vi "Check_Conn-s_bet-n_Displ_in_Track_Group-2.vi"(4 "error IN":errorcluster, 5 "[IN] # of Unconne\ncted Problem points":i32, 6 "[IN] #of Frames":i32, 7 "[IN] Clusters for Re\nconstructed Tracks":T1) -> (0 "error OUT":errorcluster, 1 "[OUT] # of Unconne\ncted Problem points":i32, 3 "[OUT] Clusters for Re\nconstructed Tracks":T1)   [LabVIEW 2017]
doc: "This subVI corrects sometimes appearing inaccuracy: appearing of points signed as problem ones but haven't any other connected points with they. The subVI just decrease of statuses of such points"
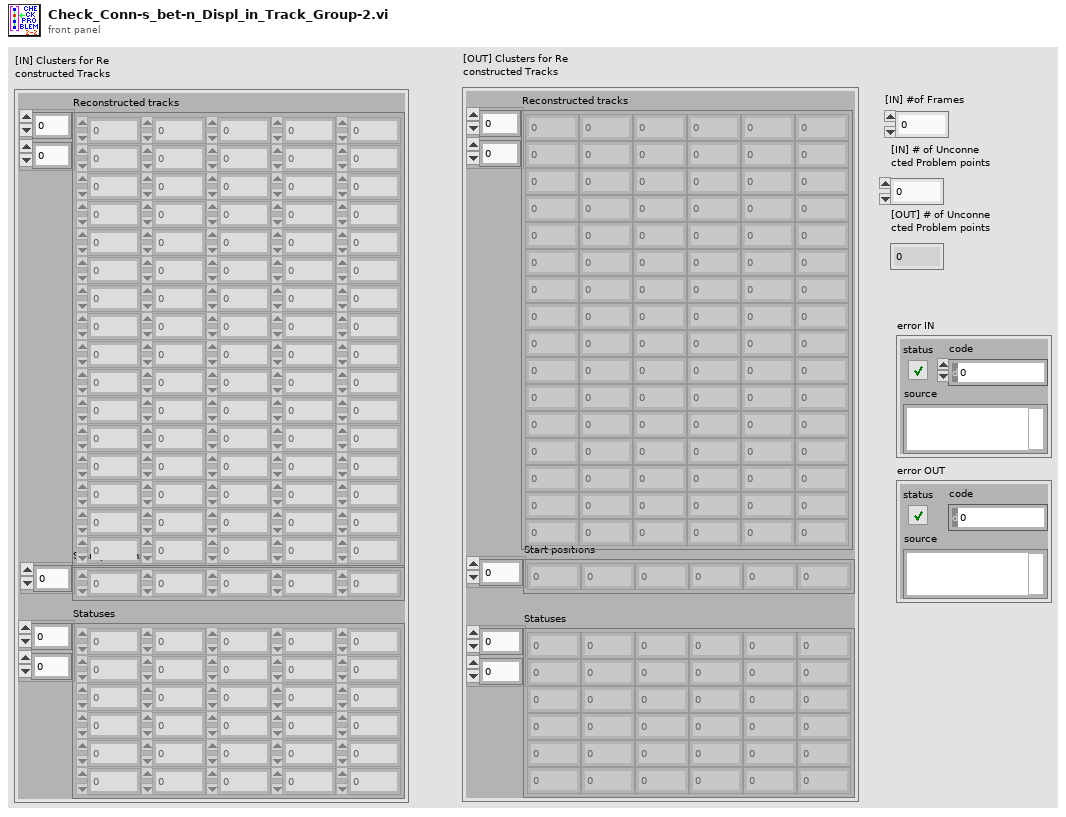
[diagram p1: front panel]
types:
  T1 = cluster{"Reconstructed tracks":dbl[][], "Start positions":i32[], "Statuses":i16[][]}
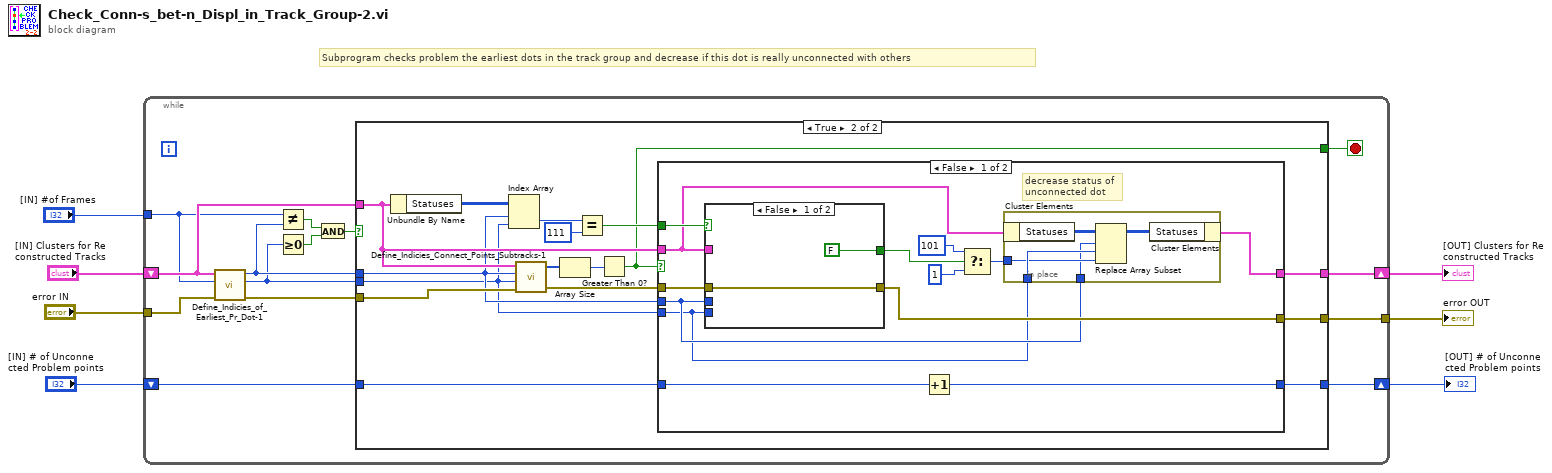
[diagram p0: block diagram]
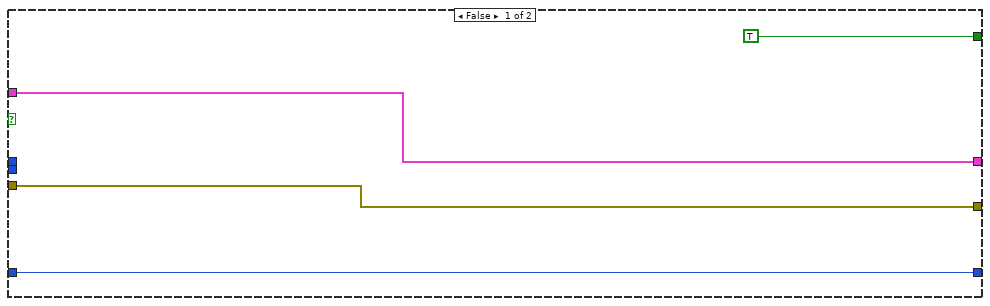
[diagram p2: hidden frame]
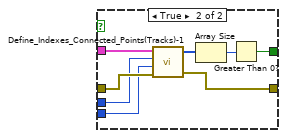
[diagram p3: hidden frame]
diagram:
  # "Subprogram checks problem the earliest dots in the track group and decrease if this dot is really unconnected with others"
  n1 = while {
    shift-right: [w17] -> w3
    shift-left: "[IN] Clusters for Re\nconstructed Tracks" -> [w18]
    tunnel: "error IN" -> [w21]
    shift-right: [w16] -> w5
    shift-left: "[IN] # of Unconne\ncted Problem points" -> [w19]
    tunnel: "[IN] #of Frames" -> [w14]
    tunnel: [w15] -> w1
    stop <- w8 stop-if-true
    n2 = call "Define_Indicies_of_Earliest_Pr_Dot-1.vi"("error IN"=w21, "[IN] #of Frames"=w14, "[IN] Still connected\ntracks in group"=w18) -> ("error OUT"=w20:errorcluster, "[OUT] Index of Subtrack"=w12:i32, "[OUT] Index of Ear\nliest Problem Point"=w13:i32)  [unwired: 2 in]
    n3 = Not Equal?(x=w14, y=w13) -> (x != y?=w10:bool)
    n4 = Greater Or Equal To 0?(x=w12) -> (x >= 0?=w9:bool)
    n5 = And(x=w10, y=w9) -> (x .and. y?=w11:bool)
    n6 = case shown="True" w11 {
      tunnel: w20 -> [w25 w41]
      tunnel: w19 -> [w24 w40]
      tunnel: w18 -> [w23 w39]
      tunnel: w13 -> [_ w37]
      tunnel: w12 -> [_ w36]
      tunnel: [w23 w29] -> w17
      tunnel: [w24 w28] -> w16
      tunnel: [w25 w27] -> w15
      tunnel: [TRUE w26] -> w8
      frame False {
      }
      frame True {
        n7 = Unbundle By Name(w39) -> ("Statuses"=w38:i16[][])
        n8 = Index Array(array=w38, index (row)=w37, index (col)=w36) -> (element=w35:i16)
        n9 = call "Define_Indicies_Connect_Points_Subtracks-1.vi"("error IN"=w41, "[IN] Index of track with\n(problem displacement)"=w36, "[IN] Index of problem\ndisplacement inside track"=w37, "[IN] Track group"=w39) -> ("error OUT"=w32:errorcluster, "[OUT] Index of connected\ntracks with problem dot"=w33:i32[])  [unwired: 1 out]
        n10 = Array Size(array=w33) -> (size(s)=w34:i32)
        n11 = Equal?(x=w35, y=i16 111) -> (x = y?=w30:bool)
        n12 = Greater Than 0?(x=w34) -> (x > 0?=w26:bool)
        n13 = case shown="False" w26 {
          tunnel: w39 -> [w46 w72]
          tunnel: [w45 w72] -> w29
          tunnel: w40 -> [w48 w70]
          tunnel: [w47 w70] -> w28
          tunnel: w37 -> [w43 _]
          tunnel: w36 -> [w42 _]
          tunnel: w32 -> [w53 w71]
          tunnel: [w52 w71] -> w27
          tunnel: w30 -> [w54 _]
          frame False {
            # "decrease status of \nunconnected dot"
            n14 = case shown="False" w54 {
              tunnel: w46 -> [_ w69]
              tunnel: w53 -> [w60 w68]
              tunnel: w43 -> [_ w67]
              tunnel: w42 -> [_ w66]
              tunnel: [FALSE w63] -> w51
              tunnel: [w60 w62] -> w52
              frame False {
              }
              frame True {
                n15 = call "Define_Indexes_Connected_Points(Tracks)-1.vi"("error IN"=w68, "[IN] Index of track with\n(problem displacement)"=w66, "[IN]Index of problem\ndisplacement inside track"=w67, "[IN] Track group"=w69) -> ("error OUT"=w62:errorcluster, "[OUT] Index of connected\ntracks with problem dot"=w64:i32[])  [unwired: 1 out]
                n16 = Array Size(array=w64) -> (size(s)=w65:i32)
                n17 = Greater Than 0?(x=w65) -> (x > 0?=w63:bool)
              }
            }
            n18 = Increment(x=w48) -> (x+1=w47:i32)
            n19 = Select(t=i16 101 ("new element/subarray"), s=w51, f=i16 1 ("new element/subarray")) -> (s? t:f=w44:i16)
            n20 = in-place {
              in-place-border: w42 -> [w57]
              in-place-border: w44 -> [w56]
              in-place-border: w43 -> [w55]
              n21 = in-place-cluster #1(w46) -> ("Statuses"=w59:i16[][])
              n22 = Replace Array Subset(array=w59, new element=w56, index (row)=w55, index (col)=w57) -> (w58:i16[][])
              n23 = in-place-cluster #1("Statuses"=w58) -> (w45:T1)
            }
          }
          frame True {
          }
        }
      }
    }
  }
  "error OUT" <- w1
  "[OUT] # of Unconne\ncted Problem points" <- w5
  "[OUT] Clusters for Re\nconstructed Tracks" <- w3
